vi "Get Volts.vi"(8 "error in (no error)":errorcluster, 11 "Osciloscopio in":refnum<class "Osciloscopio.lvclass">) -> (0 "error out":errorcluster, 2 "Volts":dbl, 3 "Osciloscopio out":refnum<class "Osciloscopio.lvclass">)   [LabVIEW 2020, in "Osciloscopio.lvclass"]
uses:
  Osciloscopio.lvclass
  Osciloscopio.lvclass/Osciloscopio.ctl
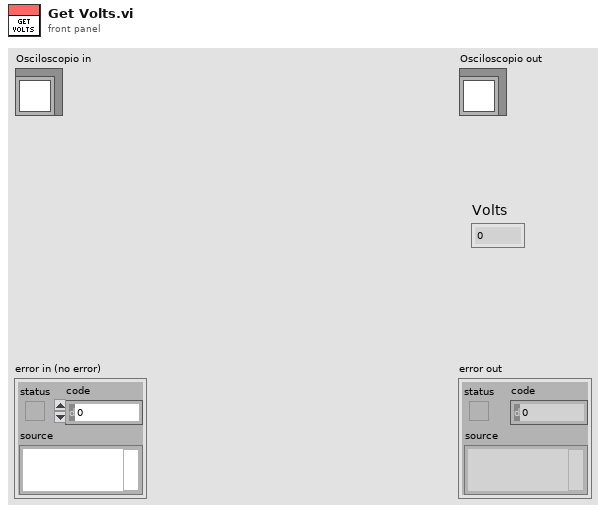
[diagram p1: front panel]
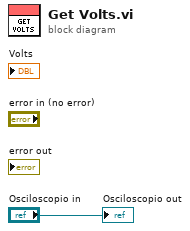
[diagram p0: block diagram]
diagram:
  "Osciloscopio out" <- "Osciloscopio in"
